vi "get db last update time.vi"(8 "error in":errorcluster, 10 "test_num":i32, 11 "conn":u32) -> (2 "field_value":string, 3 "PQresultStatus":T1(ring))   [LabVIEW 2018]
uses:
  PostgreSQL2LabVIEW/libpqlv/libpqlv.lvlib
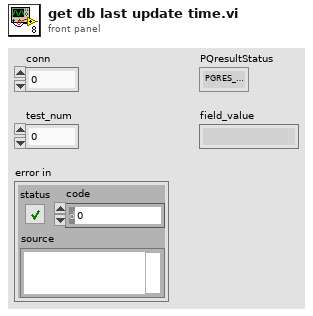
[diagram p1: front panel]
types:
  T1 = enum16{"PGRES_EMPTY_QUERY", "PGRES_COMMAND_OK", "PGRES_TUPLES_OK", "PGRES_COPY_OUT", "PGRES_COPY_IN", "PGRES_BAD_RESPONSE", "PGRES_NONFATAL_ERROR", "PGRES_FATAL_ERROR"}
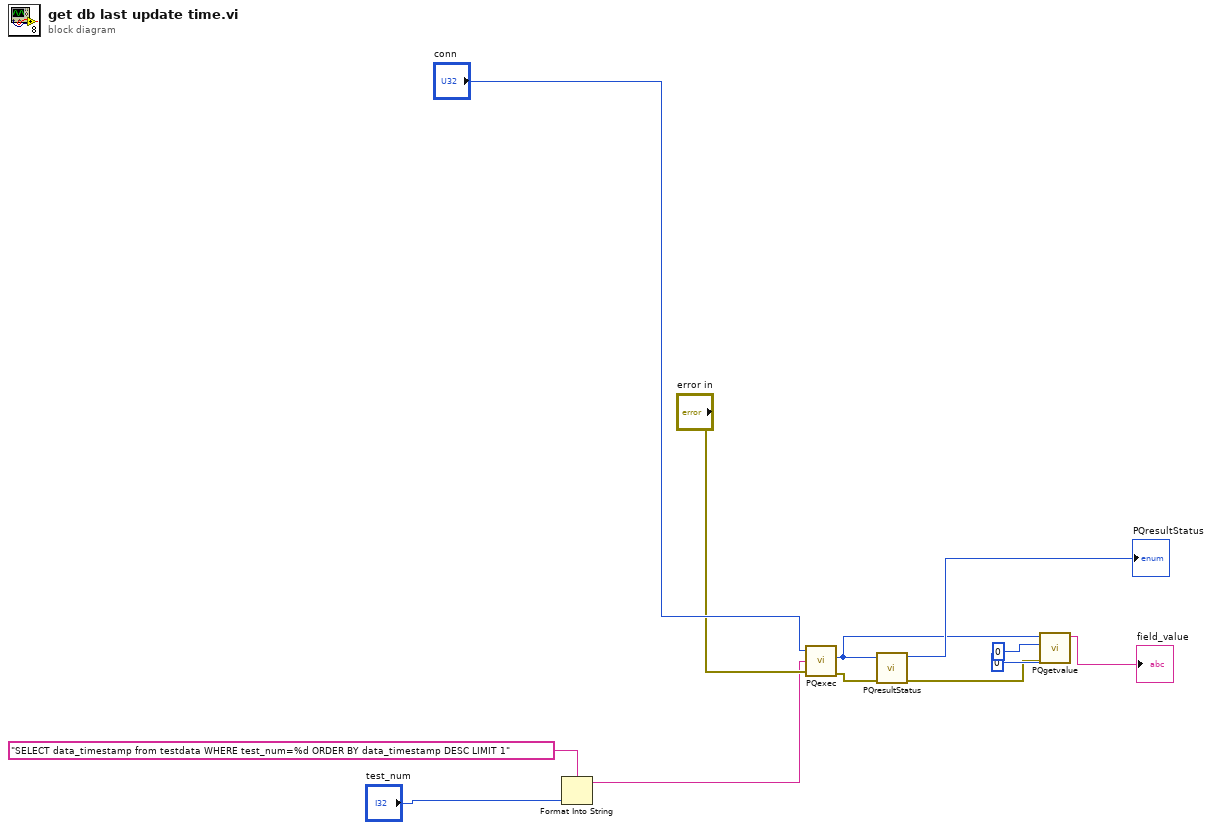
[diagram p0: block diagram]
diagram:
  n1 = Format Into String(format string="SELECT data_timestamp from testdata WHERE test_num=%d ORDER BY data_timestamp DESC LIMIT 1", "test_num") -> (resulting string=w1:string)  [unwired: 2 in, 1 out]
  n2 = call "PQexec.vi"("conn"="conn", "query"=w1, "error in (no error)"="error in") -> ("PGresult"=w2:u32, "error out"=w3:errorcluster)  [unwired: 2 in]
  n3 = call "PQresultStatus.vi"("error in (no error)"=w3, "res"=w2) -> ("error out"=w5:errorcluster, "PQresultStatus"=→"PQresultStatus":T1)  [unwired: 8 in]
  n4 = call "PQgetvalue.vi"("error in (no error)"=w5, "column_number"=0, "row_number"=0, "res"=w2) -> ("field_value"=→"field_value":string)  [unwired: 6 in, 1 out]
